vi "_Destroy.vi"(8 "error in (no error)":errorcluster, 11 "DAQmx Analog in":refnum<class "DAQmx Analog.lvclass">) -> (0 "error out":errorcluster)   [LabVIEW 2012, in "DAQmx Analog.lvclass"]
uses:
  DAQmx Analog.lvclass
  Utility Classes/Readable/Readable.lvclass
  DAQmx Analog.lvclass/DAQmx Analog.ctl
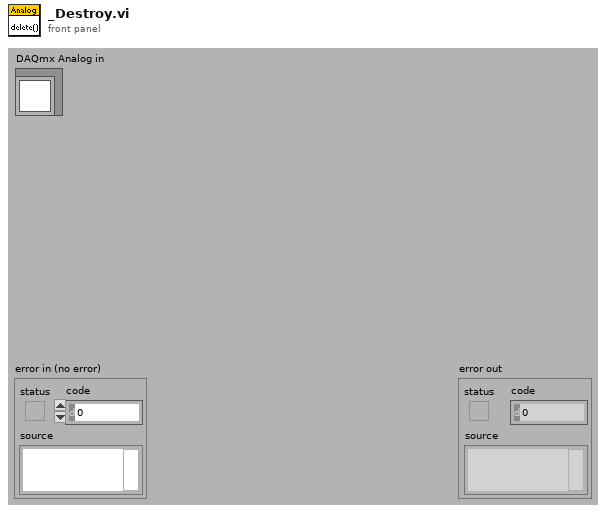
[diagram p1: front panel]
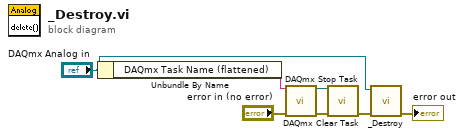
[diagram p0: block diagram]
diagram:
  n1 = Unbundle By Name("DAQmx Analog in") -> ("DAQmx Task Name (flattened)"=w7:string)
  n2 = call <vilib>:"DAQmx Stop Task.vi"("task/channels in"=w7, "error in"="error in (no error)") -> ("task out"=w5:refnum<k21>, "error out"=w3:errorcluster)  [unwired: 12 out]
  n3 = call <vilib>:"DAQmx Clear Task.vi"("task in"=w5, "error in"=w3) -> ("error out"=w6:errorcluster)  [unwired: 13 out]
  n4 = call-parent "_Destroy.vi"("error in (no error)"=w6, "Instrument in"="DAQmx Analog in") -> ("error out"=→"error out":errorcluster)  [unwired: 9 in]
